vi "SCLN_GlobalNotif.vi"(2 "Notif Write":refnum<notifier>, 3 "Element":i32 min=0 max=99, 4 "Operation":i32 min=0 max=1, 5 "Number of elements":i32=1 min=1 max=100) -> (0 "Notif Array Out":refnum<notifier>[](array[refnum]), 1 "Notif Read":refnum<notifier>)   [LabVIEW 2015]
doc: "Handle Notifier Globals Style II.\nThe globals are maintained in an uninitialized\nshift register, as an array of notifiers.\nIt is mandatory to initialize the array to\nthe number of notifiers it will contain. This\nis done on the first invocation.\n\nINPUTS:\n Operation: 1 = WRITE, 0 = READ\n Element: Element of the array to write or read\n Notif Write: Notifier to store\n\nOUTPUTS:\n Notif Read: Notifier value retrieved\n Notif Array Out: The entire array of notifiers"
panel:
  # "1 = Write"
  # "0 = Read"
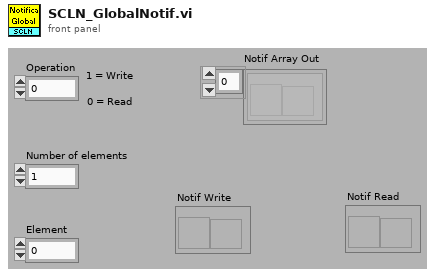
[diagram p1: front panel]
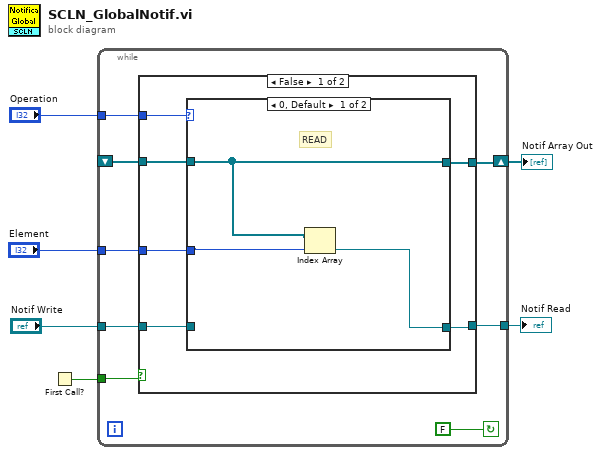
[diagram p0: block diagram]
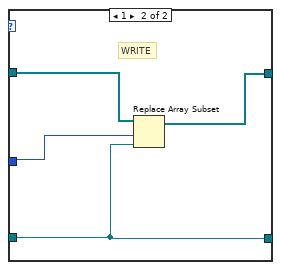
[diagram p2: hidden frame]
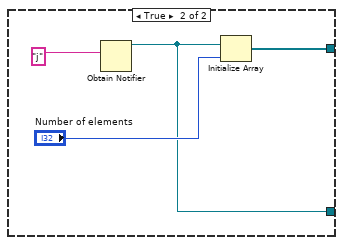
[diagram p3: hidden frame]
diagram:
  n1 = First Call?() -> (First Call?: T/F=w6:bool)
  n2 = while {
    tunnel: w6 -> [w13]
    tunnel: "Operation" -> [w12]
    tunnel: "Element" -> [w11]
    tunnel: "Notif Write" -> [w10]
    tunnel: [w9] -> w2
    shift-right: [w8] -> w1
    shift-left: _ -> [w7]
    stop <- FALSE continue-if-true
    n3 = case shown="False" w13 {
      tunnel: w12 -> [w20 _]
      tunnel: w11 -> [w18 _]
      tunnel: w10 -> [w17 _]
      tunnel: [w16 w29] -> w9
      tunnel: [w15 w28] -> w8
      tunnel: w7 -> [w19 _]
      frame False {
        n4 = case shown="0, Default" w20 {
          tunnel: w19 -> [w23 w27]
          tunnel: w18 -> [w22 w26]
          tunnel: w17 -> [_ w25]
          tunnel: [w21 w25] -> w16
          tunnel: [w23 w24] -> w15
          frame 0, Default {
            # "READ"
            n5 = Index Array(array=w23, index=w22) -> (element=w21:refnum<notifier>)
          }
          frame 1 {
            # "WRITE"
            n6 = Replace Array Subset(array=w27, new element=w25, index=w26) -> (w24:refnum<notifier>[])
          }
        }
      }
      frame True {
        n7 = Obtain Notifier(notification data type="j") -> (notifier out=w29:refnum<notifier>)  [unwired: 3 in, 2 out]
        n8 = Initialize Array(w29, "Number of elements") -> (w28:refnum<notifier>[])
      }
    }
  }
  "Notif Array Out" <- w1
  "Notif Read" <- w2
